vi "Address Control.vi"(6 "Address(line)":u32, 7 "output valid?":bool, 9 "Address(frame) input in":u32, 11 "max addr":u32) -> (2 "Address(frame) input out":u32, 3 "input ready":bool)   [LabVIEW 2015]
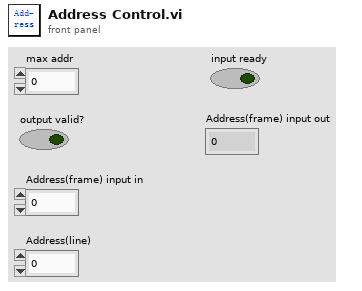
[diagram p1: front panel]
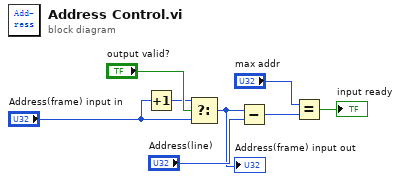
[diagram p0: block diagram]
diagram:
  n1 = Increment(x="Address(frame) input in") -> (x+1=w7:u32)
  n2 = Select(t=w7, s="output valid?", f="Address(frame) input in") -> (s? t:f=w3:u32)
  "Address(frame) input out" <- w3
  n3 = Subtract(x=w3, y="Address(line)") -> (x-y=w6:u32)
  n4 = Equal?(x="max addr", y=w6) -> (x = y?=→"input ready":bool)
